vi "DFD Nyquist Design.vi"(4 "filtering mode":T1=2 items=["No Rate Change", "Interpolation", "Decimation"], 5 "method":u16(ring)=3 items=["Kaiser Window", "Dolph-Chebyshev Window", "Equi-Ripple", "Positive Equi-Ripple"], 6 "fs in [Hz]":dbl=1.0 format="%.2f", 7 "factor":i32=4, 8 "error in (no error)":errorcluster, 9 "stopband attenuation [dB]":dbl=40.0 format="%.2f", 10 "roll off":dbl=0.2, 11 "order":i32=-1) -> (0 "error out":errorcluster, 2 "order out":i32, 3 "multirate filter out":T2={"mMRate_Structure"=enum."IIR", "mMRate_Mode"=0, "mMRate_Factor"=-1, "mMRate_FIRParams"={"mMRate_FIR_H"=[], "mMRate_FIR_IsNyquist?"=FALSE, "mMRate_FIR_IsSymmetric?"=FALSE}, "mMRate_CICParams"={"mMRate_CIC_#Stage"=0, "mMRate_CIC_Lag"=0, "mMRate_CIC_Type"=enum."Lowpass"}, "mMRate_Order"=0, "mMRate_Version"="2.0", "mMRate_Comments"="", "mMRate_RationalFactor"={"mMRate_L"=-1, "mMRate_M"=-1}, "mMRate_Fs"=1.0, "mMRate_Quantized?"=FALSE, "mMRate_QFilterGain"=1.0, "mMRate_CoefWl"=16, "mMRate_Scaling"={"mMRate_ScaleByPowerOf2?"=FALSE, "mMRate_ScaleType"=enum."No Norm"}, "mMRate_InputWl"=16, "mMRate_OutputWl"=16, "mMRate_OutputMode"=enum."Truncation", "mMRate_MultMode"=enum."Truncated", "mMRate_BitPruning"=FALSE, "mMRate_GainWl"=16, "mMRate_OutputFwl"=0, "mMRate_SumIwl"=0, "mMRate_InputIwl "=16, "mMRate_SumWl"=32, "mMRate_CoefIwl"=0} {"mMRate_SumWl" min=1 max=32 step=1; "mMRate_InputIwl" min=1 max=32 step=1; "mMRate_GainWl" min=1 max=32 step=1; "mMRate_OutputWl" min=1 max=32 step=1; "mMRate_InputWl" min=1 max=32 step=1; "mMRate_CoefWl" min=1 max=32 step=1; "mMRate_Mode" items=["Default"=-1, "No Rate Change"=0, "Interpolation"=1, "Decimation"=2, "Interpolated"=3, "Rational"=4]})   [LabVIEW 2017, in "NI_DigFilterLicensed.lvlib"]
doc: "Creates a Nyquist filter using the window or equi-ripple methods with an automatic order estimation."
uses:
  <vilib>/addons/Digital Filter Design/NI_DigFilterLicensed.lvlib
  <vilib>/addons/Digital Filter Design/_Objects.llb/DFD Multirate Filter Obj.ctl
  <vilib>/addons/Digital Filter Design/_Objects.llb/DFD Multirate Mode.ctl
  <vilib>/addons/Digital Filter Design/_Objects.llb/DFD Coef Norm Type.ctl
  <vilib>/addons/Digital Filter Design/_Objects.llb/DFD Round-off Mode.ctl
  <vilib>/addons/Digital Filter Design/_Objects.llb/DFD FXP MRate Multiply Mode.ctl
  <vilib>/addons/Digital Filter Design/_Objects.llb/DFD Multirate Filtering Mode.ctl
  <vilib>/addons/Digital Filter Design/NI_DigFilter_Process.lvlib
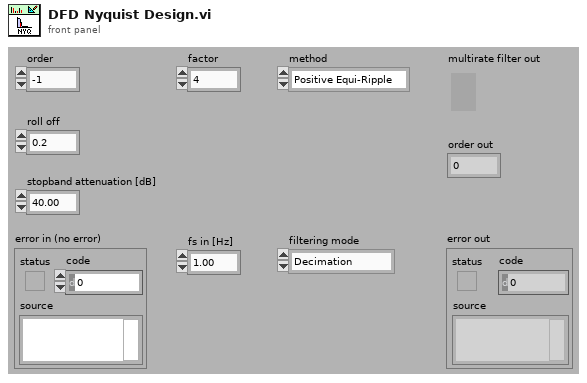
[diagram p1: front panel]
types:
  T1 = typedef "NI_DigFilterLicensed.lvlib/DFD Multirate Filtering Mode.ctl" = u16
  T2 = typedef "NI_DigFilterLicensed.lvlib/DFD Multirate Filter Obj.ctl" = cluster{"mMRate_Structure":enum16{"CIC", "FIR", "IIR", "Lattice"}, "mMRate_Mode":T3, "mMRate_Factor":i32, "mMRate_FIRParams":cluster{"mMRate_FIR_H":dbl[], "mMRate_FIR_IsNyquist?":bool, "mMRate_FIR_IsSymmetric?":bool}, "mMRate_CICParams":cluster{"mMRate_CIC_#Stage":i32, "mMRate_CIC_Lag":i32, "mMRate_CIC_Type":enum16{"Lowpass", "Highpass"}}, "mMRate_Order":i32, "mMRate_Version":string, "mMRate_Comments":string, "mMRate_RationalFactor":cluster{"mMRate_L":i32, "mMRate_M":i32}, "mMRate_Fs":dbl, "mMRate_Quantized?":bool, "mMRate_QFilterGain":dbl, "mMRate_CoefWl":i16, "mMRate_Scaling":cluster{"mMRate_ScaleByPowerOf2?":bool, "mMRate_ScaleType":T4}, "mMRate_InputWl":i16, "mMRate_OutputWl":i16, "mMRate_OutputMode":T5, "mMRate_MultMode":T6, "mMRate_BitPruning":bool, "mMRate_GainWl":i16, "mMRate_OutputFwl":i16, "mMRate_SumIwl":i16, "mMRate_InputIwl ":i16, "mMRate_SumWl":i16, "mMRate_CoefIwl":i16}
  T3 = typedef "NI_DigFilterLicensed.lvlib/DFD Multirate Mode.ctl" = i16
  T4 = typedef "NI_DigFilterLicensed.lvlib/DFD Coef Norm Type.ctl" = enum16{"No Norm", "Time Domain 1-Norm", "Time Domain 2-Norm", "Time Domain Inf-Norm"}
  T5 = typedef "NI_DigFilterLicensed.lvlib/DFD Round-off Mode.ctl" = enum16{"Nearest", "Truncation"}
  T6 = typedef "NI_DigFilterLicensed.lvlib/DFD FXP MRate Multiply Mode.ctl" = enum16{"Truncated", "Full"}
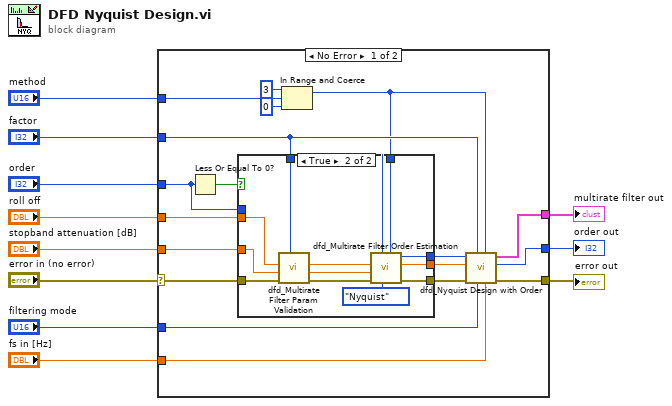
[diagram p0: block diagram]
diagram:
  n1 = case shown="No Error" "error in (no error)" {
    selector: "error in (no error)" -> [w13 w45]
    tunnel: [w29 w45] -> w11
    tunnel: "filtering mode" -> [w28 _]
    tunnel: [w27 _] -> w9
    tunnel: "factor" -> [w25 _]
    tunnel: "roll off" -> [w24 _]
    tunnel: "stopband attenuation [dB]" -> [w21 _]
    tunnel: "order" -> [w19 _]
    tunnel: "method" -> [w17 _]
    tunnel: [w14 _] -> w3
    tunnel: "fs in [Hz]" -> [w12 _]
    frame No Error {
      n2 = Less Or Equal To 0?(x=w19) -> (x <= 0?=w20:bool)
      n3 = In Range and Coerce(upper limit=u16 3, x=w17, lower limit=u16 0) -> (coerced(x)=w18:u16)  [unwired: 1 out]
      n4 = case shown="True" w20 {
        tunnel: w13 -> [w31 w44]
        tunnel: w18 -> [_ w43]
        tunnel: [w31 w41] -> w26
        tunnel: w25 -> [_ w40]
        tunnel: w24 -> [w32 w39]
        tunnel: [w30 w38] -> w23
        tunnel: [w32 w37] -> w22
        tunnel: w21 -> [_ w34]
        tunnel: w19 -> [w30 _]
        frame False {
        }
        frame True {
          n5 = call <vilib>:"dfd_Multirate Filter Param Validation.vi"("multirate factor"=w40, "error in (no error)"=w44, "A Stop [dB]"=w34, "roll off"=w39) -> ("error out"=w42:errorcluster, "dup A Stop [dB]"=w35:dbl, "dup roll off"=w36:dbl)  [unwired: 4 in, 1 out]
          n6 = call <vilib>:"dfd_Multirate Filter Order Estimation.vi"("method"=w43, "band option"=enum16{"Normal", "Nyquist", "Alias free"}."Nyquist", "multirate factor"=w40, "error in (no error)"=w42, "A Stop [dB]"=w35, "roll off"=w36) -> ("error out"=w41:errorcluster, "dup roll off"=w37:dbl, "new order"=w38:i32)  [unwired: 1 in, 2 out]
        }
      }
      n7 = call <vilib>:"dfd_Nyquist Design with Order.vi"("fs in [Hz]"=w12, "method"=w18, "filtering mode"=w28, "multirate factor"=w25, "error in (no error)"=w26, "roll off"=w22, "order"=w23) -> ("error out"=w29:errorcluster, "order out"=w27:i32, "multirate filter out"=w14:T2)  [unwired: 2 out]
    }
    frame Error {
    }
  }
  "error out" <- w11
  "multirate filter out" <- w3
  "order out" <- w9
